vi "Cal xy.vi"(0 "reference in":refnum<class "Add.lvclass">, 5 "error in (no error)":errorcluster) -> (14 "reference out":refnum<class "Add.lvclass">, 15 "result":dbl, 19 "error out":errorcluster)   [LabVIEW 2013, in "Add.lvclass"]
uses:
  Add.lvclass
  Operation_class/Operation.lvclass
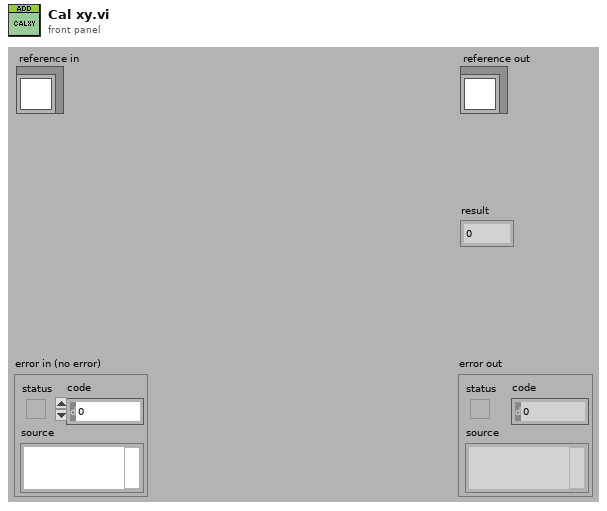
[diagram p1: front panel]
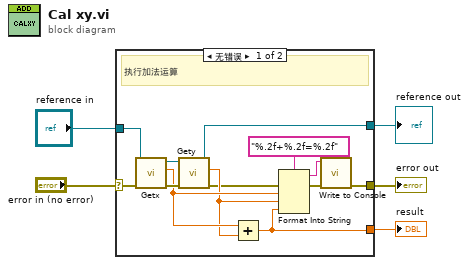
[diagram p0: block diagram]
diagram:
  n1 = case shown="无错误" "error in (no error)" {
    selector: "error in (no error)" -> [w15 w20]
    tunnel: [w7 w20] -> w4
    tunnel: [w16 w19] -> w2
    tunnel: "reference in" -> [w18 w19]
    tunnel: [w10 _] -> w1
    frame No Error {
      # "执行加法运算"
      n2 = call "Getx.vi"("error in (no error)"=w15, "reference in"=w18) -> ("error out"=w14:errorcluster, "x"=w12:dbl, "reference out"=w17:refnum<class "Add.lvclass">)  [unwired: 7 in]
      n3 = call "Gety.vi"("error in (no error)"=w14, "reference in"=w17) -> ("error out"=w8:errorcluster, "y"=w11:dbl, "reference out"=w16:refnum<class "Add.lvclass">)  [unwired: 7 in]
      n4 = Add(x=w12, y=w11) -> (x+y=w10:dbl)
      n5 = Format Into String(format string="%.2f+%.2f=%.2f" ("格式字符串"), error in=w8, w12, w11, w10) -> (resulting string=w6:string, error out=w9:errorcluster)  [unwired: 1 in]
      n6 = call "Write to Console.vi"("error in (no error)"=w9, "Input"=w6) -> ("error out"=w7:errorcluster)  [unwired: 9 in]
    }
    frame Error {
    }
  }
  "error out" <- w4
  "reference out" <- w2
  "result" <- w1
